vi "Write Solvent Solution Table.vi"(8 "Error In":errorcluster, 11 "Database Full Information In":T1 {"Database Write Information"."Layer Information Array"."Deposition Method" items=["Blade Coating", "Spin Coating", "Thermal Evaporation", "E-Beam Evaporation", "Sputtering", "Drop Casting", "Dip Coating", "Pulsed Laser Deposition", "Chemival Vapour Deposition", "Atomic Layer Deposition", "Spray Coating", "Screen Printing", "Electroplating", "Molecular Beam Epitaxy", "Custom Deposition"]; "Database Write Information"."Layer Information Array"."Layer Type" items=["Front Electrode", "Electron Transport Layer", "Active Layer", "Hole Transport Layer", "Back Electrode", "Custom Layer"]}) -> (0 "Error Out":errorcluster, 3 "Database Full Information Out":T1 {"Database Write Information"."Layer Information Array"."Deposition Method" items=["Blade Coating", "Spin Coating", "Thermal Evaporation", "E-Beam Evaporation", "Sputtering", "Drop Casting", "Dip Coating", "Pulsed Laser Deposition", "Chemival Vapour Deposition", "Atomic Layer Deposition", "Spray Coating", "Screen Printing", "Electroplating", "Molecular Beam Epitaxy", "Custom Deposition"]; "Database Write Information"."Layer Information Array"."Layer Type" items=["Front Electrode", "Electron Transport Layer", "Active Layer", "Hole Transport Layer", "Back Electrode", "Custom Layer"]})   [LabVIEW 2020]
uses:
  Data Clusters/Database Information.ctl
  Data Clusters/Layer Information Cluster.ctl
  <vilib>/addons/database/Connection.llb/Conn ObjectReference.ctl
  <vilib>/addons/database/NI_Database_API.lvlib
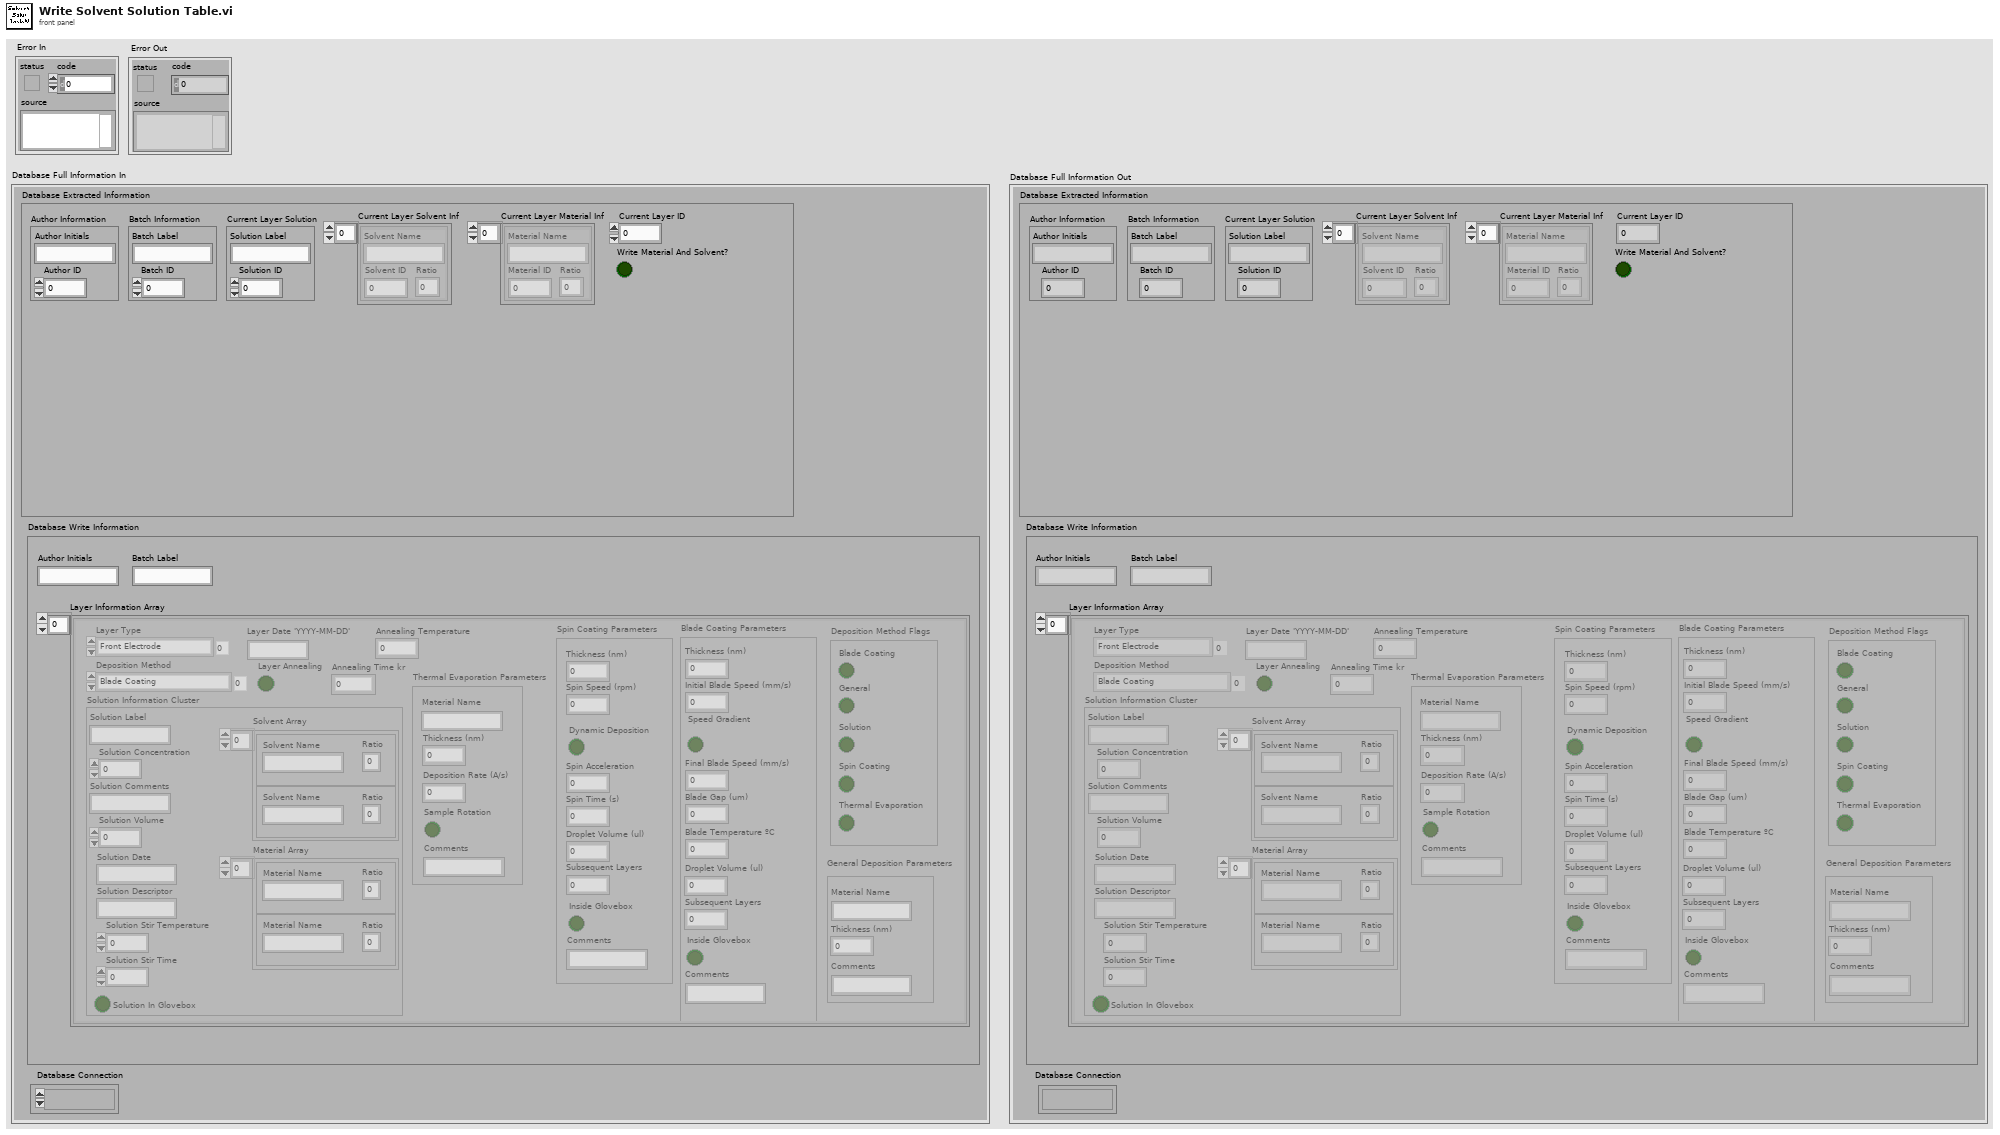
[diagram p1: front panel]
types:
  T1 = typedef "Database Information.ctl" = cluster{"Database Extracted Information":cluster{"Author Information":cluster{"Author Initials":string, "Author ID":i32}, "Batch Information":cluster{"Batch Label":string, "Batch ID":i32}, "Current Layer Solution":cluster{"Solution Label":string, "Solution ID":i32}, "Current Layer ID":i32, "Current Layer Solvent Inf":cluster{"Solvent Name":string, "Solvent ID":i32, "Ratio":dbl}[], "Current Layer Material Inf":cluster{"Material Name":string, "Material ID":i32, "Ratio":dbl}[], "Write Material And Solvent?":bool}, "Database Write Information":cluster{"Author Initials":string, "Batch Label":string, "Layer Information Array":T2[]}, "Database Connection":T3}
  T2 = typedef "Layer Information Cluster.ctl" = cluster{"Solution Information Cluster":cluster{"Solution Label":string, "Solution Concentration":dbl, "Solution Comments ":string, "Solution Volume ":dbl, "Solution Date ":string, "Solution Descriptor ":string, "Solution Stir Temperature ":dbl, "Solution Stir Time ":dbl, "Solution In Glovebox":bool, "Solvent Array":cluster{"Solvent Name":string, "Ratio":dbl}[], "Material Array":cluster{"Material Name":string, "Ratio":dbl}[]}, "Layer Type":u16, "Deposition Method":u16, "Layer Annealing":bool, "General Deposition Parameters":cluster{"Thickness (nm)":dbl, "Comments":string, "Material Name":string}, "Blade Coating Parameters":cluster{"Thickness (nm)":dbl, "Initial Blade Speed (mm/s)":dbl, "Speed Gradient":bool, "Final Blade Speed (mm/s)":dbl, "Blade Gap (um)":dbl, "Droplet Volume (ul)":dbl, "Subsequent Layers":dbl, "Inside Glovebox":bool, "Comments":string, "Blade Temperature ºC":dbl}, "Spin Coating Parameters":cluster{"Thickness (nm)":dbl, "Spin Speed (rpm)":dbl, "Dynamic Deposition":bool, "Spin Acceleration":dbl, "Spin Time (s)":dbl, "Droplet Volume (ul)":dbl, "Subsequent Layers":dbl, "Inside Glovebox":bool, "Comments":string}, "Thermal Evaporation Parameters":cluster{"Deposition Rate (A/s)":dbl, "Thickness (nm)":dbl, "Comments":string, "Material Name":string, "Sample Rotation":bool}, "Layer Date 'YYYY-MM-DD'":string, "Annealing Time kr":dbl, "Annealing Temperature":dbl, "Deposition Method Flags":cluster{"Blade Coating":bool, "General ":bool, "Solution":bool, "Spin Coating":bool, "Thermal Evaporation":bool}}
  T3 = typedef "NI_Database_API.lvlib/Conn ObjectReference.ctl" = refnum<k1>
  T4 = cluster{"Solvent Name":string, "Solvent ID":i32, "Ratio":dbl}[]
  T5 = cluster{"Solution ID":i32, "Solvent ID":i32, "Ratio":dbl}
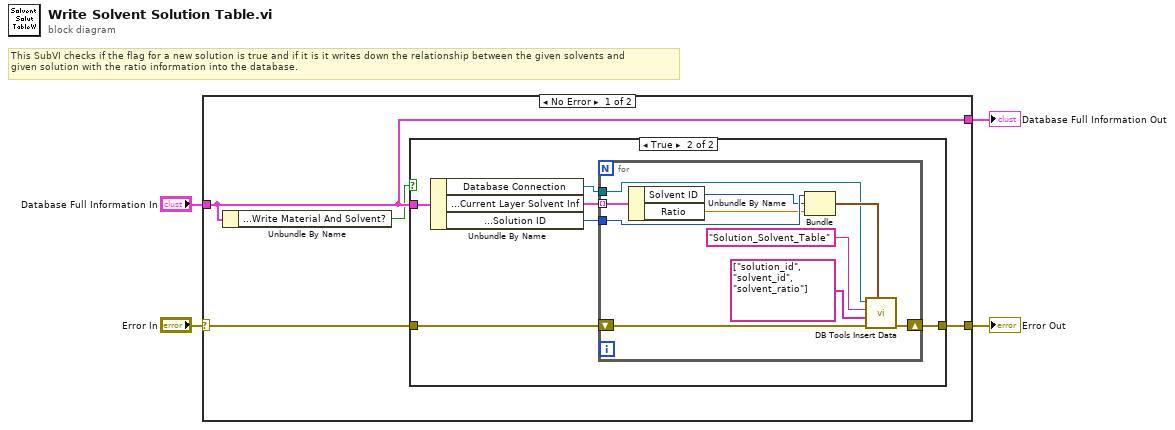
[diagram p0: block diagram]
diagram:
  # "This SubVI checks if the flag for a new solution is true and if it is it writes down the relationship between the given solvents and \ngiven solution with the ratio information into the database."
  n1 = case shown="No Error" "Error In" {
    selector: "Error In" -> [w8 w27]
    tunnel: [w7 w27] -> w3
    tunnel: "Database Full Information In" -> [w6 w26]
    tunnel: [w6 w26] -> w1
    frame No Error {
      n2 = Unbundle By Name(w6) -> ("Database Extracted Information.Write Material And Solvent?"=w5:bool)
      n3 = case shown="True" w5 {
        tunnel: w8 -> [w9 w15]
        tunnel: [w9 w14] -> w7
        tunnel: w6 -> [_ w10]
        frame False {
        }
        frame True {
          n4 = Unbundle By Name(w10) -> ("Database Connection"=w13:T3, "Database Extracted Information.Current Layer Solvent Inf"=w12:T4, "Database Extracted Information.Current Layer Solution.Solution ID"=w11:i32)
          n5 = for {
            tunnel: w13 -> [w19]
            shift-right: [w16] -> w14
            shift-left: w15 -> [w18]
            tunnel: w12 -> [w25] mode=indexing
            tunnel: w11 -> [w23]
            n6 = Unbundle By Name(w25) -> ("Solvent ID"=w22:i32, "Ratio"=w21:dbl)
            n7 = Bundle("Solution ID"=w23, "Solvent ID"=w22, "Ratio"=w21) -> (w20:T5)  [unwired: 1 in]
            n8 = call <vilib>:"DB Tools Insert Data.vi"("data"=w20, "error in (no error)"=w18, "columns"=string[] ["solution_id", "solvent_id", "solvent_ratio"], "table"="Solution_Solvent_Table", "connection reference"=w19) -> ("error out"=w16:errorcluster)  [unwired: 5 in, 1 out]
          }
        }
      }
    }
    frame Error {
    }
  }
  "Error Out" <- w3
  "Database Full Information Out" <- w1
